vi "Traffic Light.vi"() -> ()   [LabVIEW 2015]
panel:
  in  "Start":bool
  out "?":bool
  out "?":bool
  out "?":bool
  in  "Pause":bool
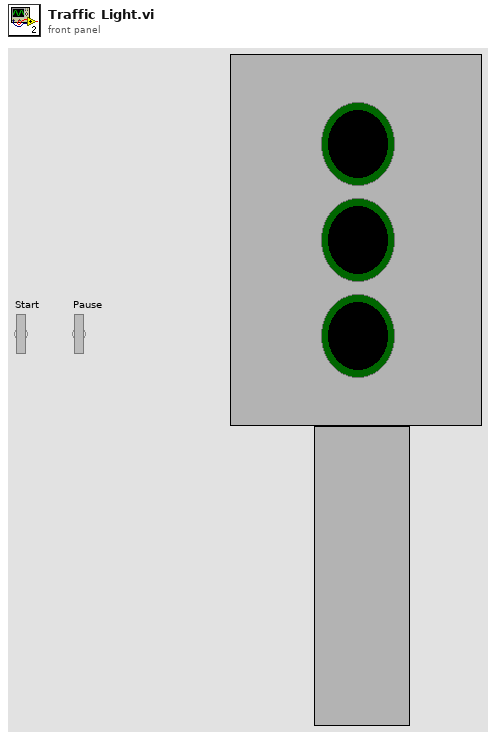
[diagram p1: front panel]
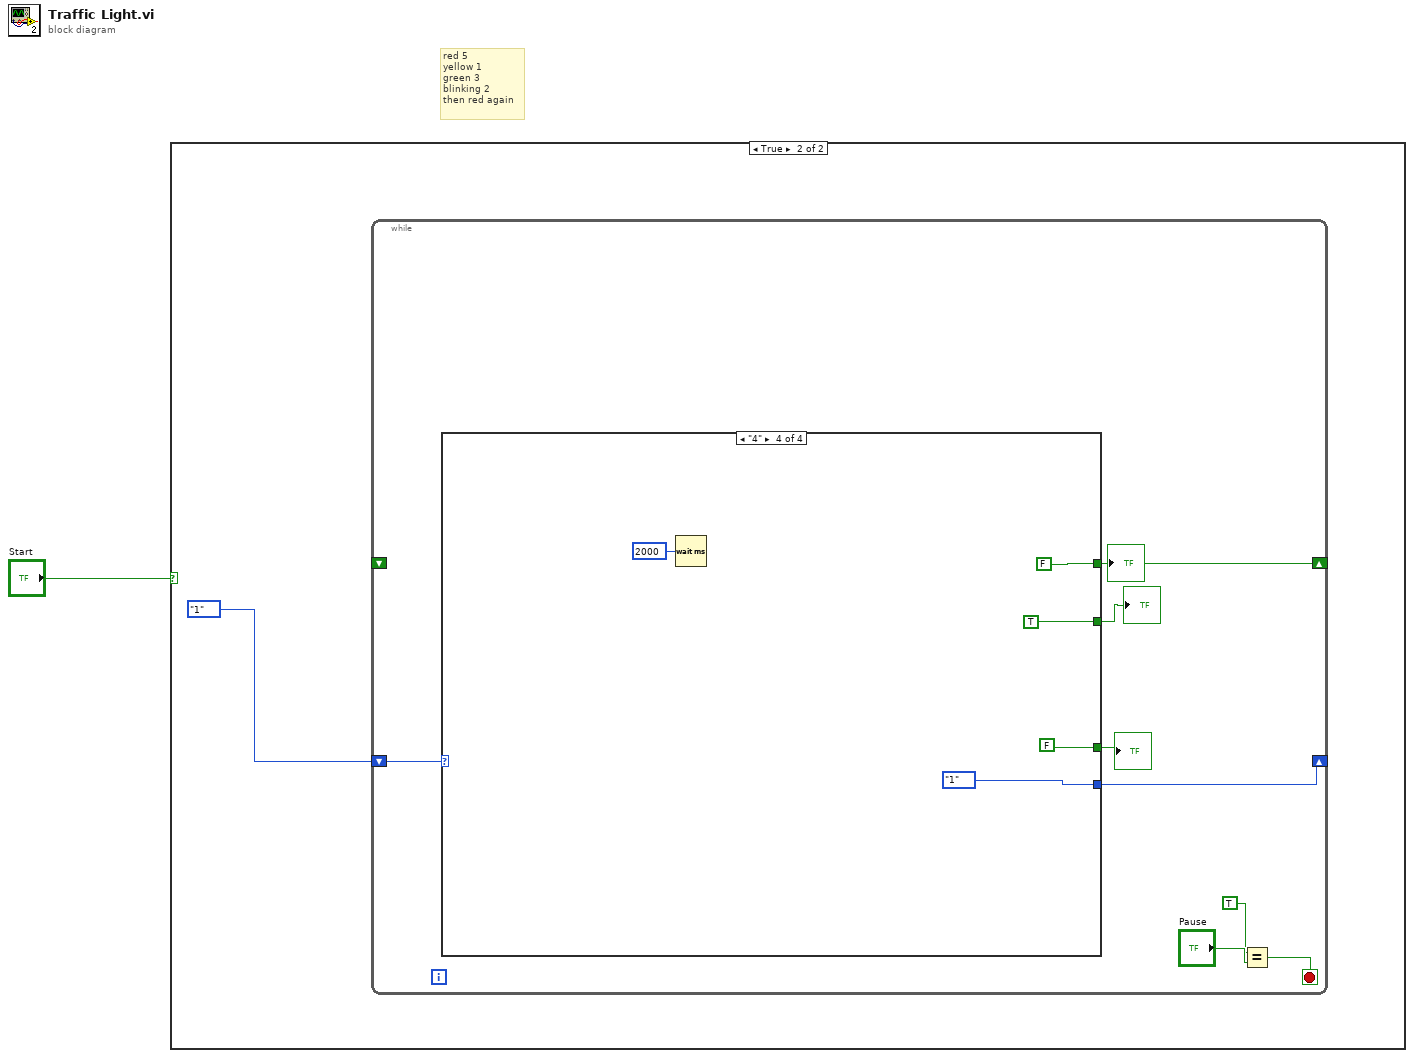
[diagram p0: block diagram]
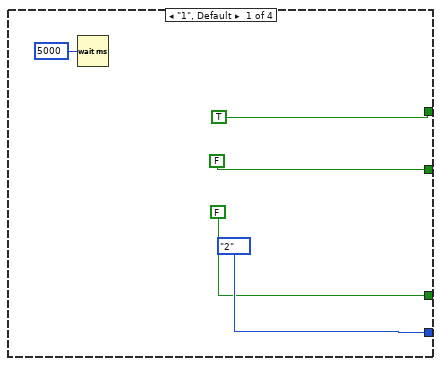
[diagram p3: hidden frame]
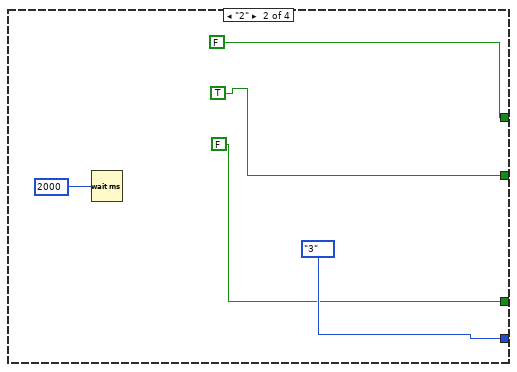
[diagram p4: hidden frame]
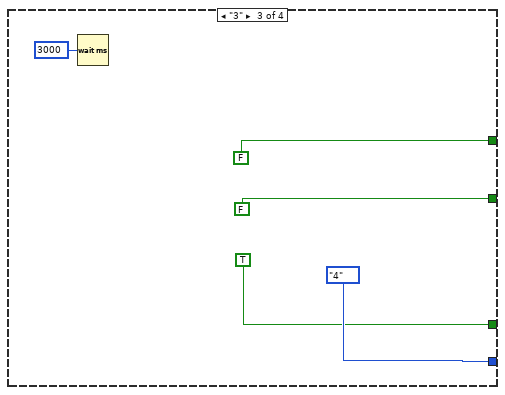
[diagram p5: hidden frame]
diagram:
  # "red 5\nyellow 1\ngreen 3\nblinking 2\nthen red again"
  n1 = case shown="True" "Start" {
    frame False {
    }
    frame True {
      n2 = while {
        shift-right: [w9] -> _
        shift-left: enum16{"1", "2", "3", "4", ""}."1" -> [w10]
        shift-right: [w4] -> _
        shift-left: _ -> [_]
        stop <- w6 stop-if-true
        n3 = case shown="\"4\"" w10 {
          tunnel: [enum16{"1", "2", "3", "4", ""}."2" enum16{"1", "2", "3", "4", ""}."3" enum16{"1", "2", "3", "4", ""}."4" enum16{"1", "2", "3", "4", ""}."1"] -> w9
          tunnel: [FALSE FALSE TRUE FALSE] -> w5
          tunnel: [TRUE FALSE FALSE FALSE] -> w4
          tunnel: [FALSE TRUE FALSE TRUE] -> w3
          frame "1", Default {
            n4 = Wait (ms)(milliseconds to wait=u32 5000) -> ()  [unwired: 1 out]
          }
          frame "2" {
            n5 = Wait (ms)(milliseconds to wait=u32 2000) -> ()  [unwired: 1 out]
          }
          frame "3" {
            n6 = Wait (ms)(milliseconds to wait=u32 3000) -> ()  [unwired: 1 out]
          }
          frame "4" {
            n7 = Wait (ms)(milliseconds to wait=u32 2000) -> ()  [unwired: 1 out]
          }
        }
        "?" <- w3
        "?" <- w4
        "?" <- w5
        n8 = Equal?(x=TRUE, y="Pause") -> (x = y?=w6:bool)
      }
    }
  }
